vi "GenerateCode.vi"(0 "XRef":T10, 1 "Terms":T7, 2 "Diagram":T6, 3 "State In":T1) -> (14 "Generated Code?":T5, 15 "Reply":T3, 16 "Fatal Error Out":T2, 17 "State Out":T1)   [LabVIEW 2015, in "Index JSON Array.xnode"]
uses:
  Index JSON Array.xnode
  <vilib>/XNodeSupport/XNodeXNodeRef.ctl
  <vilib>/XNodeSupport/XNodeTermIDPairs.ctl
  <vilib>/XNodeSupport/XNodeTermIDPair.ctl
  <vilib>/XNodeSupport/XNodeTermRef.ctl
  <vilib>/XNodeSupport/XNodeString.ctl
  <vilib>/XNodeSupport/XNodeTopLevelDiagramRef.ctl
  State.ctl
  <vilib>/XNodeSupport/XNodeBool.ctl
  <vilib>/XNodeSupport/XNodeStringArray.ctl
  <vilib>/XNodeSupport/XNodeErrorCluster.ctl
  <vilib>/Utility/miscctls.llb/LVPointTypeDef.ctl
  Index Array.vi
  <vilib>/XNodeSupport/NI_XNodeSupport.lvlib
  JSON Array.lvclass
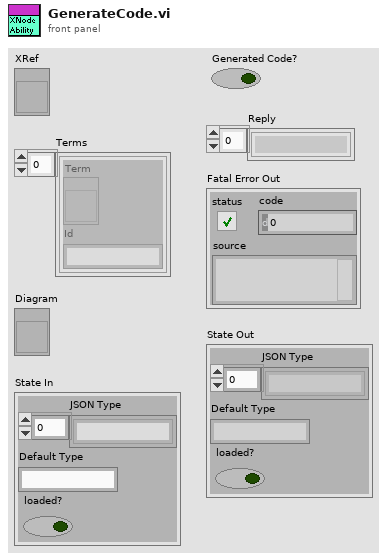
[diagram p1: front panel]
types:
  T1 = typedef "Index JSON Array.xnode/State.ctl" = cluster{"JSON Type":string[], "Default Type":string, "loaded?":bool}
  T2 = typedef "NI_XNodeSupport.lvlib/XNodeErrorCluster.ctl" = errorcluster
  T3 = typedef "NI_XNodeSupport.lvlib/XNodeStringArray.ctl" = T4[]
  T4 = typedef "NI_XNodeSupport.lvlib/XNodeString.ctl" = string
  T5 = typedef "NI_XNodeSupport.lvlib/XNodeBool.ctl" = bool
  T6 = typedef "NI_XNodeSupport.lvlib/XNodeTopLevelDiagramRef.ctl" = refnum<vi>
  T7 = typedef "NI_XNodeSupport.lvlib/XNodeTermIDPairs.ctl" = T8[]
  T8 = typedef "NI_XNodeSupport.lvlib/XNodeTermIDPair.ctl" = cluster{"Term":T9, "Id":T4}
  T9 = typedef "NI_XNodeSupport.lvlib/XNodeTermRef.ctl" = refnum<vi>
  T10 = typedef "NI_XNodeSupport.lvlib/XNodeXNodeRef.ctl" = refnum<vi>
  T11 = typedef "LVPointTypeDef.ctl" = cluster{"Horizontal":i16, "Vertical":i16}
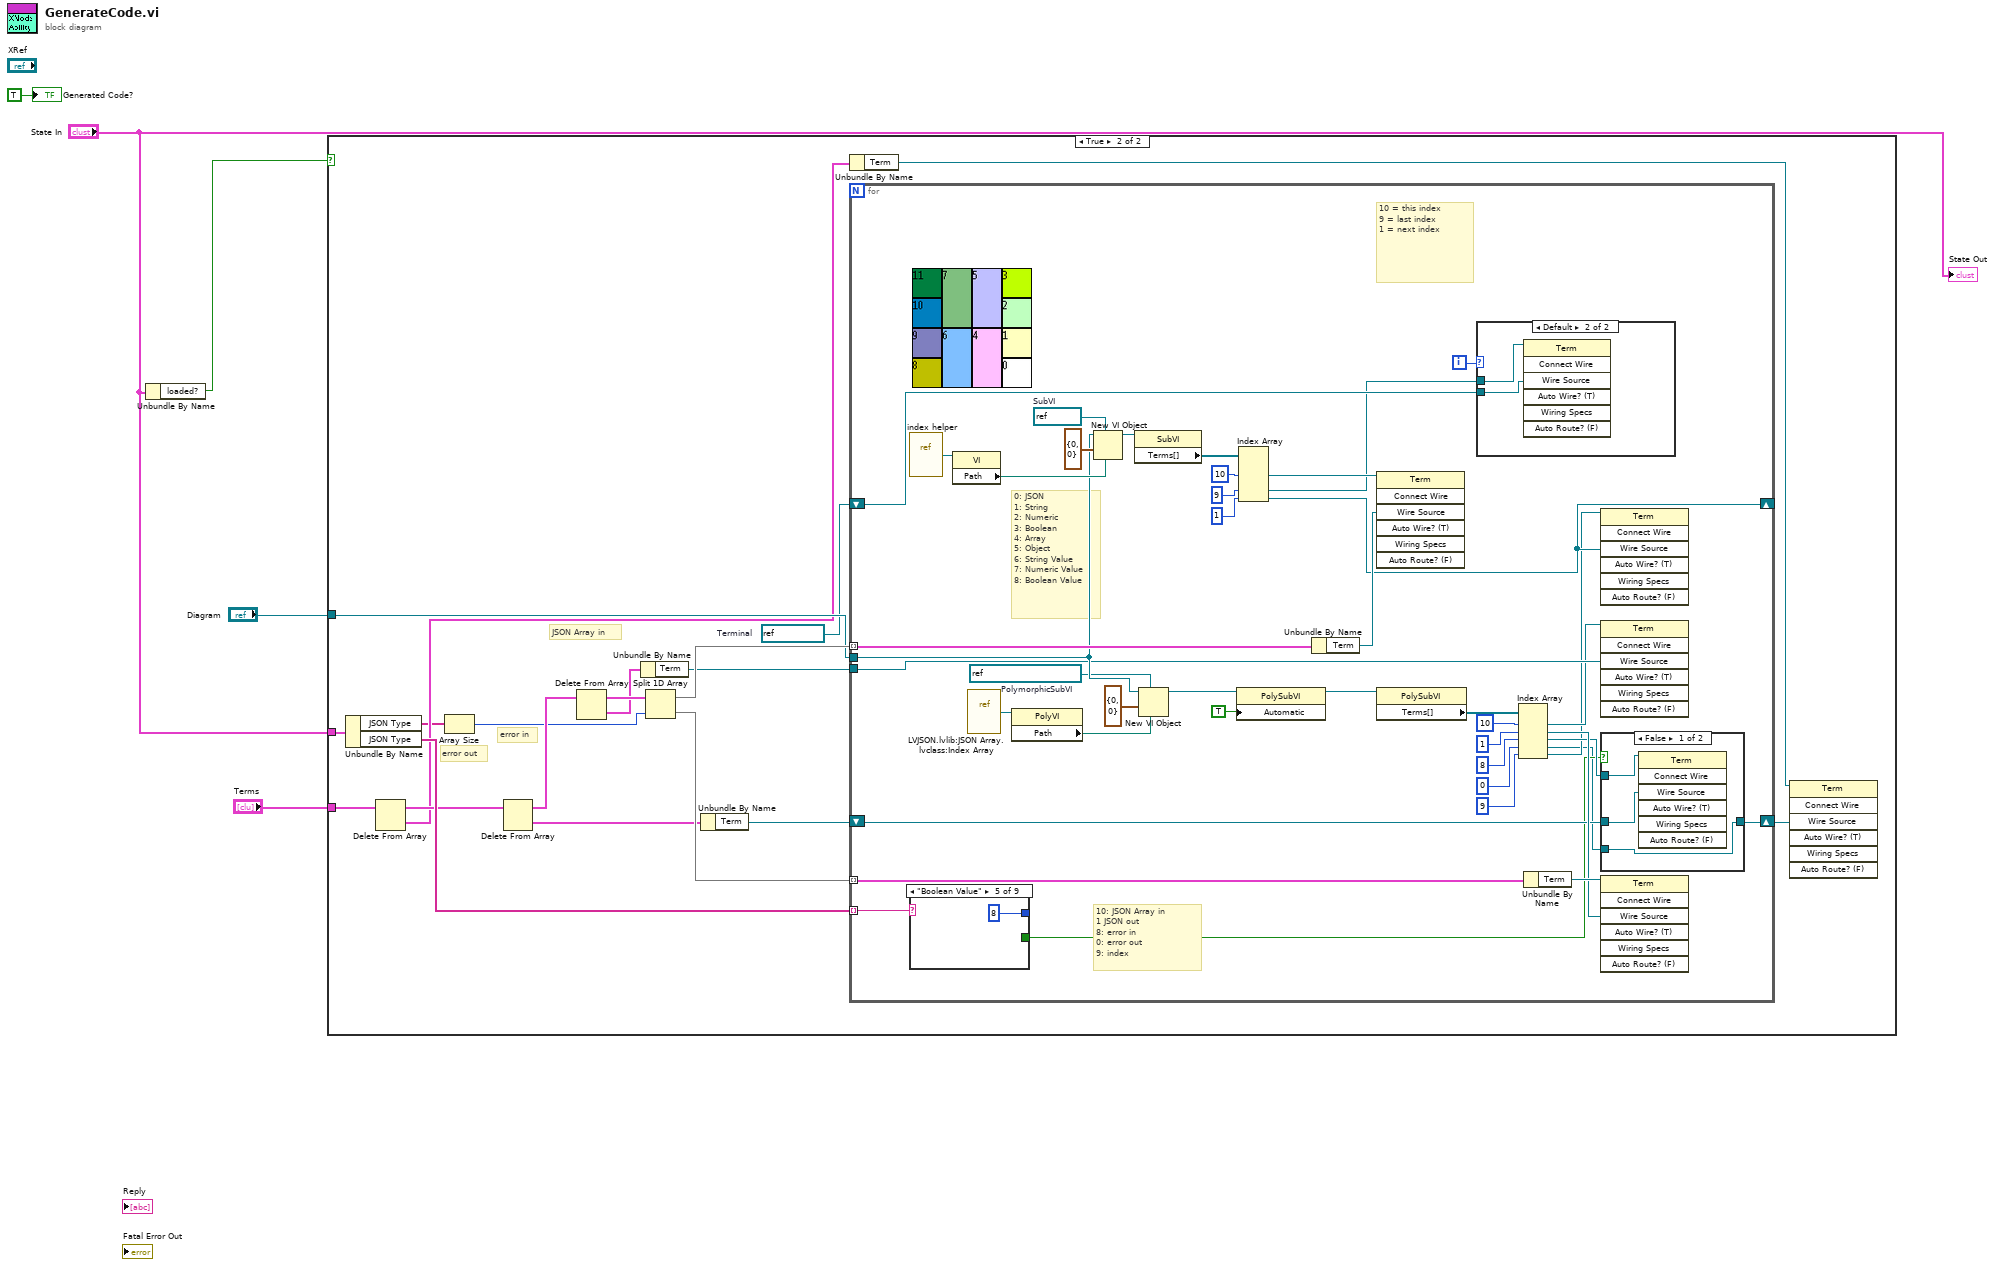
[diagram p0: block diagram]
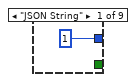
[diagram p4: hidden frame]
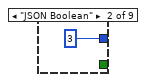
[diagram p5: hidden frame]
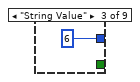
[diagram p6: hidden frame]
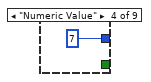
[diagram p7: hidden frame]
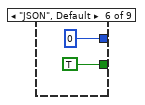
[diagram p8: hidden frame]
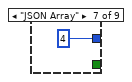
[diagram p9: hidden frame]
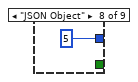
[diagram p10: hidden frame]
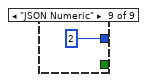
[diagram p11: hidden frame]
diagram:
  n1 = Unbundle By Name("State In") -> ("loaded?"=w1:bool)
  n2 = case shown="True" w1 {
    tunnel: "State In" -> [_ w24]
    tunnel: "Diagram" -> [_ w21]
    tunnel: "Terms" -> [_ w15]
    frame False {
    }
    frame True {
      w17 = refnum<vi> refnum  # Terminal
      # "JSON Array in"
      # "error in"
      # "error out"
      n3 = Unbundle By Name(w24) -> ("JSON Type"=w7:string[], "JSON Type"=w16:string[])
      n4 = Delete From Array(array=w15) -> (deleted portion=w12:T8, array with subset deleted=w14:T7)  [unwired: 2 in]
      n5 = Array Size(array=w7) -> (size(s)=w6:i32)
      n6 = Delete From Array(array=w14) -> (deleted portion=w11:T8, array with subset deleted=w13:T7)  [unwired: 2 in]
      n7 = Delete From Array(array=w13) -> (deleted portion=w19:T8, array with subset deleted=w20:T7)  [unwired: 2 in]
      n8 = Unbundle By Name(w19) -> ("Term"=w18:T9)
      n9 = Split 1D Array(array=w20, index=w6) -> (first subarray=w23:T7, second subarray=w22:T7)
      n10 = Unbundle By Name(w11) -> ("Term"=w10:T9)
      n11 = Unbundle By Name(w12) -> ("Term"=w9:T9)
      n12 = for {
        tunnel: w23 -> [w57] mode=indexing
        tunnel: w22 -> [w58] mode=indexing
        tunnel: w21 -> [w48]
        tunnel: w18 -> [w45]
        shift-right: [w44] -> _
        shift-left: w17 -> [w55]
        tunnel: w16 -> [w50] mode=indexing
        shift-right: [w27] -> w8
        shift-left: w10 -> [w46]
        i -> [w53]
        w39 = refnum<vi> refnum  # PolymorphicSubVI
        w65 = refnum<vi> refnum  # SubVI
        # "10: JSON Array in\n1 JSON out\n8: error in\n0: error out\n9: index"
        # "0: JSON\n1: String\n2: Numeric\n3: Boolean\n4: Array\n5: Object\n6: String Value\n7: Numeric Value\n8: Boolean Value"
        # "10 = this index\n9 = last index\n1 = next index"
        n13 = vi-ref "index helper.vi"() -> (w63:refnum<vi>)
        n14 = case shown="\"Boolean Value\"" w50 {
          tunnel: [1 ("Selected Type") 3 ("Selected Type") 6 ("Selected Type") 7 ("Selected Type") 8 ("Selected Type") 0 ("Selected Type") 4 ("Selected Type") 5 ("Selected Type") 2 ("Selected Type")] -> _
          tunnel: [_ _ _ _ _ TRUE _ _ _] -> w28
          frame "JSON String" {
          }
          frame "JSON Boolean" {
          }
          frame "String Value" {
          }
          frame "Numeric Value" {
          }
          frame "Boolean Value" {
          }
          frame "JSON", Default {
          }
          frame "JSON Array" {
          }
          frame "JSON Object" {
          }
          frame "JSON Numeric" {
          }
        }
        n15 = property class="VI"(reference=w63) -> ("Path"=w64:path)  [unwired: 1 in, 2 out]
        n16 = vi-ref "LVJSON.lvlib:JSON Array.lvclass:Index Array.vi"() -> (w36:refnum<vi>)
        n17 = property class="PolyVI"(reference=w36) -> ("Path"=w38:path)  [unwired: 1 in, 2 out]
        n18 = New VI Object(vi object class=w65, owner refnum=w48, position/next to=T11 {"Horizontal"=0, "Vertical"=0} ("location"), 6:w64) -> (object refnum=w62:refnum<vi>)  [unwired: 4 in, 1 out]
        n19 = property class="SubVI"(reference=w62) -> ("Terms[]"=w61:refnum<vi>[])  [unwired: 1 in, 2 out]
        n20 = New VI Object(vi object class=w39, owner refnum=w48, position/next to=T11 {"Horizontal"=0, "Vertical"=0} ("location"), 6:w38) -> (object refnum=w37:refnum<vi>)  [unwired: 4 in, 1 out]
        n21 = property class="PolySubVI"(reference=w37, "Automatic"=TRUE) -> (reference out=w41:refnum<vi>)  [unwired: 1 in, 1 out]
        n22 = Index Array(array=w61, index #2=10 ("index"), index #4=9 ("index"), index #5=1 ("index")) -> (element #2=w59:refnum<vi>, element #4=w54:refnum<vi>, element #5=w44:refnum<vi>)  [unwired: 2 in, 2 out]
        n23 = Unbundle By Name(w57) -> ("Term"=w56:T9)
        n24 = invoke class="Term" method="Connect Wire"(reference=w59, "Wire Source"=w56) -> ()  [unwired: 5 in, 7 out]
        n25 = property class="PolySubVI"(reference=w41) -> ("Terms[]"=w42:refnum<vi>[])  [unwired: 1 in, 2 out]
        n26 = case shown="Default" w53 {
          tunnel: w55 -> [_ w82]
          tunnel: w54 -> [_ w81]
          frame 0 {
          }
          frame Default {
            n27 = invoke class="Term" method="Connect Wire"(reference=w81, "Wire Source"=w82) -> ()  [unwired: 5 in, 7 out]
          }
        }
        n28 = Index Array(array=w42, index #1=10 ("index"), index #2=1 ("index"), index #3=8 ("index"), index #4=0 ("index"), index #5=9 ("index")) -> (element #1=w34:refnum<vi>, element #2=w47:refnum<vi>, element #3=w31:refnum<vi>, element #4=w26:refnum<vi>, element #5=w29:refnum<vi>)
        n29 = Unbundle By Name(w58) -> ("Term"=w49:T9)
        n30 = invoke class="Term" method="Connect Wire"(reference=w29, "Wire Source"=w44) -> ()  [unwired: 5 in, 7 out]
        n31 = invoke class="Term" method="Connect Wire"(reference=w34, "Wire Source"=w45) -> ()  [unwired: 5 in, 7 out]
        n32 = case shown="False" w28 {
          tunnel: w46 -> [w69 w70]
          tunnel: w31 -> [w68 _]
          tunnel: [w67 w70] -> w27
          tunnel: w26 -> [w67 _]
          frame False {
            n33 = invoke class="Term" method="Connect Wire"(reference=w68, "Wire Source"=w69) -> ()  [unwired: 5 in, 7 out]
          }
          frame True {
          }
        }
        n34 = invoke class="Term" method="Connect Wire"(reference=w49, "Wire Source"=w47) -> ()  [unwired: 5 in, 7 out]
      }
      n35 = invoke class="Term" method="Connect Wire"(reference=w9, "Wire Source"=w8) -> ()  [unwired: 5 in, 7 out]
    }
  }
  "Generated Code?" <- T5 TRUE ("Generated Code?")
  "State Out" <- "State In"
